vi "Fit Model to Raw Plot.vi"(6 "Termination Criteria":T1={"Max Iterations"=1000, "Max Function Calls"=10000, "Max Time"=1000.0, "Function Tolerance"=1e-06, "Parameter Tolerance"=1e-06, "Gradient Tolerance"=1e-06, "Min Lambda"=1e-06, "Max Lambda"=1000000.0, "Initial Tick Count"=0}, 7 "Fit Settings":T3 {"Confidence Level" min=0.0 max=100.0; "Axis Type" items=["Linear", "Logarithmic"]}, 8 "error in (no error)":errorcluster, 9 "Fit Model Information":T9, 10 "Plot Name (Plot)":string="Plot", 11 "Plot":T2) -> (0 "error out":errorcluster, 1 "Fit Output Data":T11, 2 "Array of Plots (Fit, n Components, Residuals)":cluster{"X Array":dbl[], "Y Array":dbl[]}[](array[cluster]), 3 "Fit Output Arrays":T12, 4 "Fit Plot Name":string, 5 "Residual Type":string)   [LabVIEW 2021, in "Fits.lvlib"]
doc: "Takes a <B>Plot</B> and fits it to the specified model."
uses:
  Fits.lvlib
  Fit Output Data.ctl
  Fit Output Arrays.ctl
  Fit Models.ctl
  Fit Model Information.ctl
  Nonlinear Fit Method.ctl
  Ramp Type.ctl
  Residual Type.ctl
  Non-linear Fitting Algorithm.ctl
  Fit Settings.ctl
  Graphs/XY Graph/XY Graph Plot Data.ctl
  Graphs/XY Graph/XY Graph Add-Ons.lvlib
  My Fit Stopping Criteria.ctl
  IRF(X)PSED/Fit Weights Type v2.ctl
panel:
  # "see the License on the block diagram (Ctrl+E or Window:Show Block Diagram)"
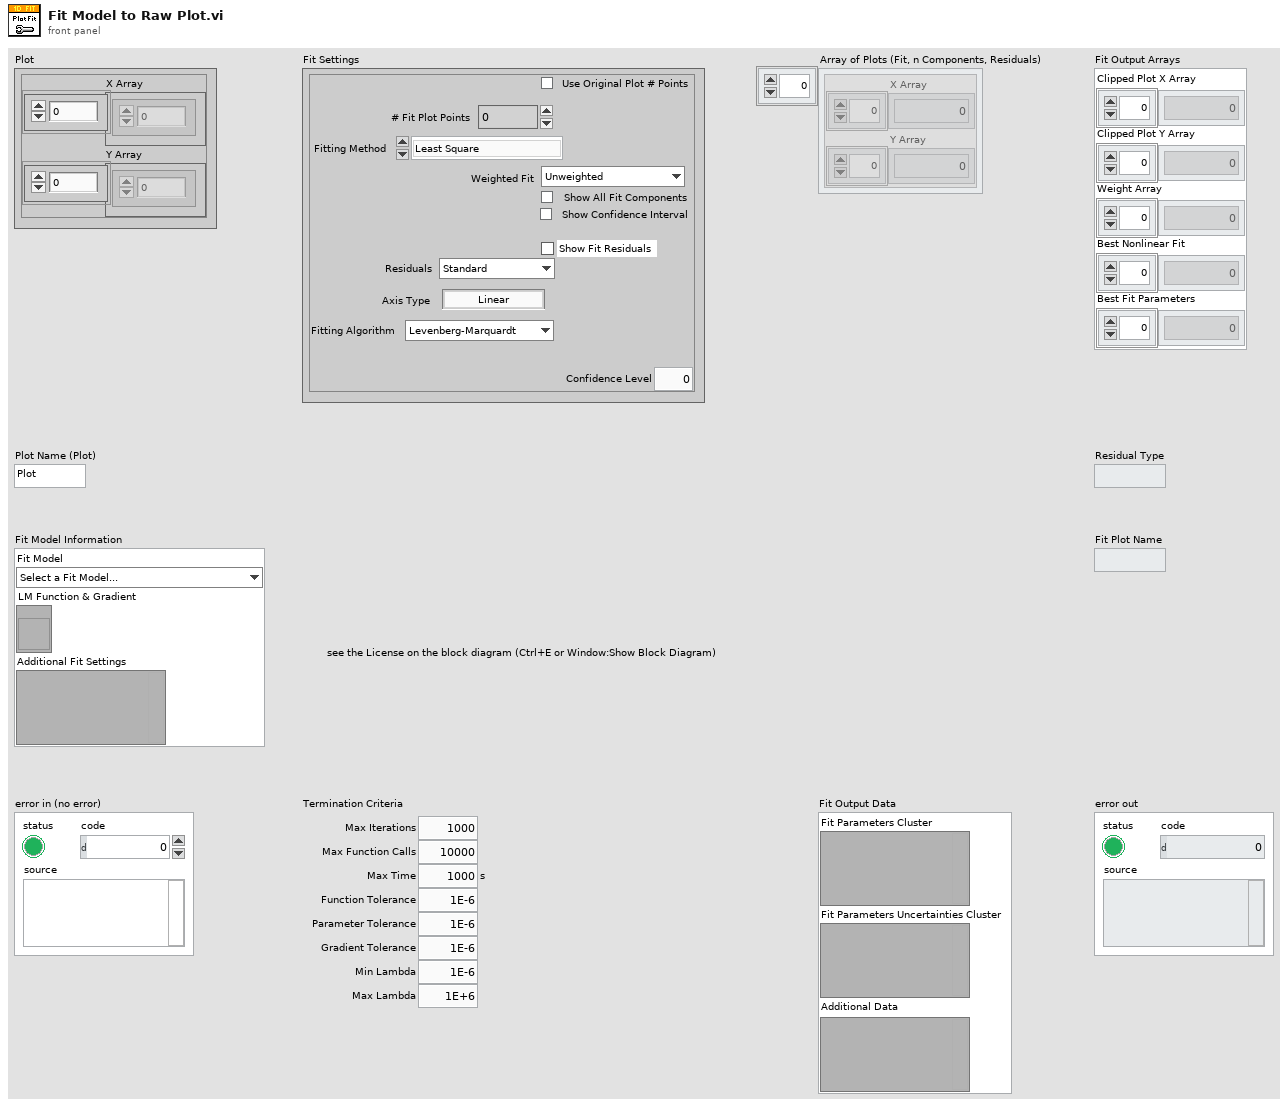
[diagram p1: front panel]
types:
  T1 = typedef "Fits.lvlib/My Fit Stopping Criteria.ctl" = cluster{"Max Iterations":i32, "Max Function Calls":i32, "Max Time":dbl[unit], "Function Tolerance":dbl, "Parameter Tolerance":dbl, "Gradient Tolerance":dbl, "Min Lambda":dbl, "Max Lambda":dbl, "Initial Tick Count":u32}
  T2 = typedef "XY Graph Add-Ons.lvlib/XY Graph Plot Data.ctl" = cluster{"X Array":dbl[], "Y Array":dbl[]}
  T3 = typedef "Fits.lvlib/Fit Settings.ctl" = cluster{"Use Original Plot # Points":bool, "# Fit Plot Points":u32, "Fitting Method":T4, "Weighted Fit":T5, "Show All Fit Components":bool, "Axis Type":T6, "Show Fit Residuals":bool, "Residual Type":T7, "Fitting Algorithm":T8, "Show Confidence Interval":bool, "Confidence Level":dbl}
  T4 = typedef "Fits.lvlib/Nonlinear Fit Method.ctl" = enum16{"Least Square", "Least Absolute Residual", "Bisquare", "MLE"}
  T5 = typedef "Fits.lvlib/Fit Weights Type v2.ctl" = enum16{"Unweighted", "1/Variance (Neyman)", "1/Variance (Pearson)", "Best of All"}
  T6 = typedef "Fits.lvlib/Ramp Type.ctl" = u16
  T7 = typedef "Fits.lvlib/Residual Type.ctl" = enum16{"Standard", "Normalized", "Reduced"}
  T8 = typedef "Fits.lvlib/Non-linear Fitting Algorithm.ctl" = enum16{"Levenberg-Marquardt", "Trust-Region Dogleg"}
  T9 = typedef "Fits.lvlib/Fit Model Information.ctl" = cluster{"Fit Model":T10, "LM Function & Gradient":refnum<vi>, "Additional Fit Settings":variant}
  T10 = typedef "Fits.lvlib/Fit Models.ctl" = enum16{"Select a Fit Model...", "           Single Peak", "Gaussian", "Asymmetric Gaussian", "Lorentzian", "Asymmetric Lorentzian", "Gaussian/Lorentzian", "Lorentzian/Gaussian", "           Double Peak", "Two Gaussians", "Two Asymmetric Gaussians", "Two H-Connected Gaussians", "Two T-Connected Gaussians", "Two H-Connected Asymmetric Gaussians", "Two T-Connected Asymmetric Gaussians", "           Triple Peak", "Three Gaussians", "Three Asymmetric Gaussians", "              Decays", "1-Exponential", "IRF*PSED", "2-Exponentials", "            Power Law", "Power Law", "Power Law with Offset", "               ACF", "2D Gaussian ACF", "2D Gaussian + Blinking ACF", "2D Gaussian + Flow ACF", "3D Gaussian ACF", "3D Gaussian + Blinking ACF", "             Multiplot", "2D Gaussian ACF & 2D Gaussian + Flow ACF"}
  T11 = typedef "Fits.lvlib/Fit Output Data.ctl" = cluster{"Fit Parameters Cluster":variant, "Fit Parameters Uncertainties Cluster":variant, "Additional Data":variant}
  T12 = typedef "Fits.lvlib/Fit Output Arrays.ctl" = cluster{"Clipped Plot X Array":dbl[], "Clipped Plot Y Array":dbl[], "Weight Array":dbl[], "Best Nonlinear Fit":dbl[], "Best Fit Parameters":dbl[]}
  T13 = cluster{"X Array":dbl[], "Y Array":dbl[], "Weight Array":dbl[]}
  T14 = cluster{"parameter minimum":dbl[], "parameter maximum":dbl[]}
  T15 = cluster{"best fit parameters":dbl[], "best nonlinear fit":dbl[]}
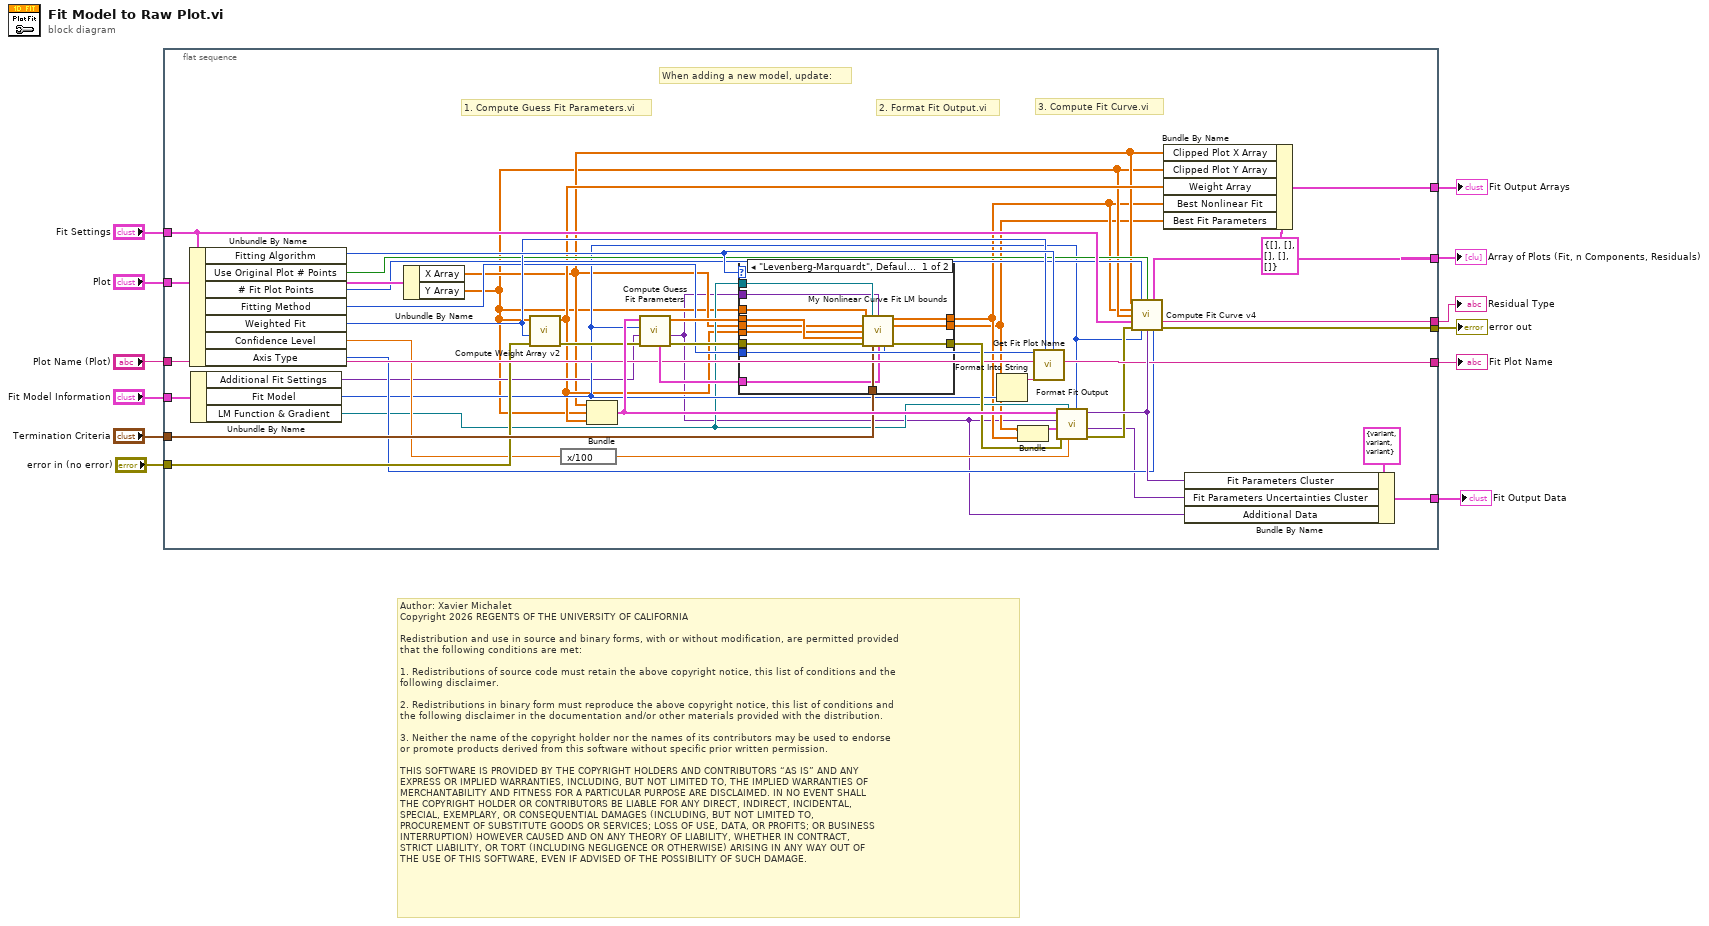
[diagram p0: block diagram]
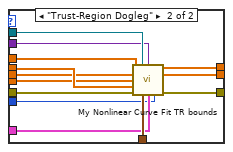
[diagram p2: hidden frame]
diagram:
  # "Author: Xavier Michalet\nCopyright 2026 REGENTS OF THE UNIVERSITY OF CALIFORNIA\n\nRedistribution and use in source and binary forms, with or without modification, are permitted provided\nthat the following conditions are met:\n\n1. Redistributions of source code must retain the above copyright notice, this list of conditions and the\nfollowing disclaimer.\n\n2. Redistributions in binary form must reproduce the above copyright notice, this list of conditions and\nthe following disclaimer in the documentation and/or other materials provided with the distribution.\n\n3. Neither the name of the copyright holder nor the names of its contributors may be used to endorse \nor promote products derived from this software without specific prior written permission.\n\nTHIS SOFTWARE IS PROVIDED BY THE COPYRIGHT HOLDERS AND CONTRIBUTORS “AS IS” AND ANY \nEXPRESS OR IMPLIED WARRANTIES, INCLUDING, BUT NOT LIMITED TO, THE IMPLIED WARRANTIES OF\nMERCHANTABILITY AND FITNESS FOR A PARTICULAR PURPOSE ARE DISCLAIMED. IN NO EVENT SHALL\nTHE COPYRIGHT HOLDER OR CONTRIBUTORS BE LIABLE FOR ANY DIRECT, INDIRECT, INCIDENTAL, \nSPECIAL, EXEMPLARY, OR CONSEQUENTIAL DAMAGES (INCLUDING, BUT NOT LIMITED TO, \nPROCUREMENT OF SUBSTITUTE GOODS OR SERVICES; LOSS OF USE, DATA, OR PROFITS; OR BUSINESS\nINTERRUPTION) HOWEVER CAUSED AND ON ANY THEORY OF LIABILITY, WHETHER IN CONTRACT, \nSTRICT LIABILITY, OR TORT (INCLUDING NEGLIGENCE OR OTHERWISE) ARISING IN ANY WAY OUT OF\nTHE USE OF THIS SOFTWARE, EVEN IF ADVISED OF THE POSSIBILITY OF SUCH DAMAGE."
  n1 = flat-sequence {
    tunnel: [w51] -> w1
    tunnel: [w50] -> w2
    tunnel: "Termination Criteria" -> [w47]
    tunnel: [w43] -> w4
    tunnel: "Plot Name (Plot)" -> [w42]
    tunnel: "Plot" -> [w41]
    tunnel: "error in (no error)" -> [w40]
    tunnel: [w38] -> w10
    tunnel: "Fit Settings" -> [w37]
    tunnel: "Fit Model Information" -> [w27]
    tunnel: [w21] -> w11
    tunnel: [w14] -> w12
    frame #0 {
      # "When adding a new model, update:"
      # "3. Compute Fit Curve.vi"
      # "2. Format Fit Output.vi"
      # "1. Compute Guess Fit Parameters.vi"
      n2 = Unbundle By Name(w37) -> ("Fitting Algorithm"=w36:T8, "Use Original Plot # Points"=w30:bool, "# Fit Plot Points"=w29:u32, "Fitting Method"=w31:T4, "Weighted Fit"=w32:T5, "Confidence Level"=w34:dbl, "Axis Type"=w35:T6)
      n3 = Unbundle By Name(w27) -> ("Additional Fit Settings"=w24:variant, "Fit Model"=w26:T10, "LM Function & Gradient"=w25:refnum<vi>)
      n4 = Unbundle By Name(w41) -> ("X Array"=w19:dbl[], "Y Array"=w18:dbl[])
      n5 = call "Compute Weight Array v2.vi"("Error In"=w40, "Weighted Fit"=w32, "Data Array"=w18) -> ("Error Out"=w39:errorcluster, "Weight Array"=w20:dbl[])  [unwired: 7 in]
      n6 = expression code="x/100"(w34) -> (w33:dbl)
      n7 = Bundle("X Array"=w19, "Y Array"=w18, "Weight Array"=w20) -> (w53:T13)  [unwired: 1 in]
      n8 = call "Compute Guess Fit Parameters.vi"("error in (no error)"=w39, "Additional Data"=w24, "Fit Model"=w26, "Data in"=w53) -> ("error out"=w49:errorcluster, "Additional LM Data"=w13:variant, "Initial Fit Parameters"=w45:dbl[], "Parameter Bounds"=w46:T14)  [unwired: 4 in]
      n9 = case shown="\"Levenberg-Marquardt\", Default" w36 {
        tunnel: w49 -> [w67 w80]
        tunnel: w47 -> [w66 w79]
        tunnel: w46 -> [w65 w78]
        tunnel: w25 -> [w64 w77]
        tunnel: w45 -> [w63 w76]
        tunnel: w20 -> [w62 w75]
        tunnel: w31 -> [w61 w74]
        tunnel: w13 -> [w60 w73]
        tunnel: w18 -> [w59 w72]
        tunnel: w19 -> [w58 w71]
        tunnel: [w57 w70] -> w17
        tunnel: [w56 w69] -> w44
        tunnel: [w55 w68] -> w16
        frame "Levenberg-Marquardt", Default {
          n10 = call "My Nonlinear Curve Fit LM bounds.vi"("Y"=w59, "f(x,a)"=w64, "data"=w60, "X"=w58, "Weight"=w62, "initial parameters"=w63, "error in (no error)"=w67, "Termination Criteria"=w66, "parameter bounds"=w65, "NL Fit Method"=w61) -> ("best nonlinear fit"=w57:dbl[], "best fit parameters"=w55:dbl[], "error out"=w56:errorcluster)  [unwired: 3 out]
        }
        frame "Trust-Region Dogleg" {
          n11 = call "My Nonlinear Curve Fit TR bounds.vi"("Y"=w72, "f(x,a)"=w77, "data"=w73, "X"=w71, "Weight"=w75, "initial parameters"=w76, "error in (no error)"=w80, "Termination Criteria"=w79, "parameter bounds"=w78, "method"=w74) -> ("best nonlinear fit"=w70:dbl[], "best fit parameters"=w68:dbl[], "error out"=w69:errorcluster)  [unwired: 3 out]
        }
      }
      n12 = Format Into String(w26) -> (resulting string=w28:string)  [unwired: 3 in, 1 out]
      n13 = Bundle("best fit parameters"=w16, "best nonlinear fit"=w17) -> (w52:T15)  [unwired: 1 in]
      n14 = call "Get Fit Plot Name.vi"("Fitting Algorithm"=w36, "Weighted Histogram Fit"=w32, "Fit Model"=w28, "Plot Name"=w42, "Fit Method"=w31) -> ("Fit Plot Name"=w51:string)  [unwired: 6 in]
      n15 = call "Format Fit Output.vi"("Fit Model"=w26, "confidence level (0.68)"=w33, "f(x,a)"=w25, "Error In"=w44, "Fit Results"=w52, "Additional Data"=w13, "Data in"=w53) -> ("Error Out"=w48:errorcluster, "Fit Parameters Uncertainties Cluster"=w22:variant, "Fit Parameters Cluster"=w54:variant)  [unwired: 2 in]
      n16 = call "Compute Fit Curve v4.vi"("X Array in"=w19, "# Points"=w29, "Use Same Number of Points as Histogram"=w30, "Best Fit in"=w17, "Y Array in"=w18, "Fit Settings"=w37, "Error In"=w48, "Fit Model"=w26, "Fit Parameters"=w54, "Ramp Type"=w35) -> ("Array of Plots (Fit, n Components, Residuals)"=w38:cluster{"X Array":dbl[], "Y Array":dbl[]}[], "Residual Type"=w43:string, "Error Out"=w50:errorcluster)  [unwired: 3 out]
      n17 = Bundle By Name(cluster=T12 {"Clipped Plot X Array"=[], "Clipped Plot Y Array"=[], "Weight Array"=[], "Best Nonlinear Fit"=[], "Best Fit Parameters"=[]}, "Clipped Plot X Array"=w19, "Clipped Plot Y Array"=w18, "Weight Array"=w20, "Best Nonlinear Fit"=w17, "Best Fit Parameters"=w16) -> (w14:T12)
      n18 = Bundle By Name(cluster=T11 {"Fit Parameters Cluster"=variant, "Fit Parameters Uncertainties Cluster"=variant, "Additional Data"=variant} ("Fit Output Data"), "Fit Parameters Cluster"=w54, "Fit Parameters Uncertainties Cluster"=w22, "Additional Data"=w13) -> (w21:T11)
    }
  }
  "Fit Output Arrays" <- w12
  "Fit Output Data" <- w11
  "Array of Plots (Fit, n Components, Residuals)" <- w10
  "Residual Type" <- w4
  "error out" <- w2
  "Fit Plot Name" <- w1
